vi "Send Message.vi"(4 "timeout in ms (100)":i32=100, 6 "Message ID":i32, 8 "error in (no error)":errorcluster, 9 "Data":variant, 10 "Command":string, 11 "RemoteControl.STM in":refnum<class "RemoteControl.STM.lvclass">) -> (0 "error out":errorcluster, 3 "RemoteControl.STM out":refnum<class "RemoteControl.STM.lvclass">)   [LabVIEW 2016, in "RemoteControl.STM.lvclass"]
uses:
  RemoteControl.STM.lvclass
  <vilib>/NI/STM/TCP/TCP Write Options.ctl
  RemoteControl/Typedefs/Variant with Message ID-cluster.ctl
  RemoteControl.STM.lvclass/RemoteControl.STM.ctl
  <vilib>/NI/STM/TCP/Write Message (TCP).vi
  <vilib>/NI/STM/NI STM.lvlib
  RemoteControl/RemoteControl.lvclass
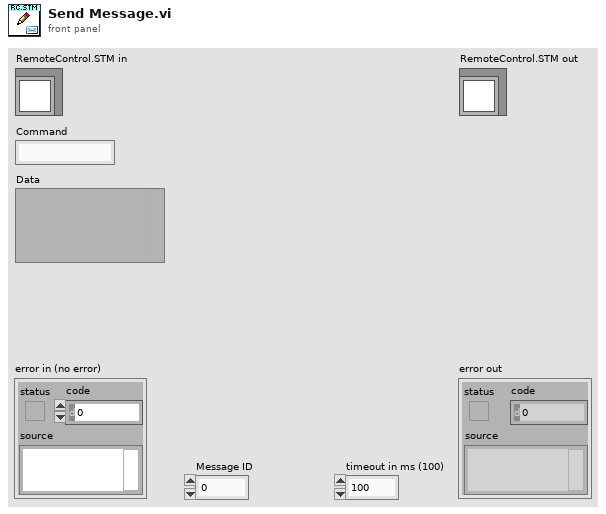
[diagram p1: front panel]
types:
  T1 = typedef "RemoteControl.lvclass/Variant with Message ID-cluster.ctl" = cluster{"Data":variant, "Message ID":i32}
  T2 = typedef "NI STM.lvlib/TCP Write Options.ctl" = cluster{"ignore timeout error":bool, "timeout ms (1000)":i32}
  T3 = typedef "NI STM.lvlib/TCP Connection Info.ctl" = cluster{"connection ID":refnum<k5>, "meta data":T4[]}
  T4 = typedef "NI STM.lvlib/MetaDataElement.ctl" = string
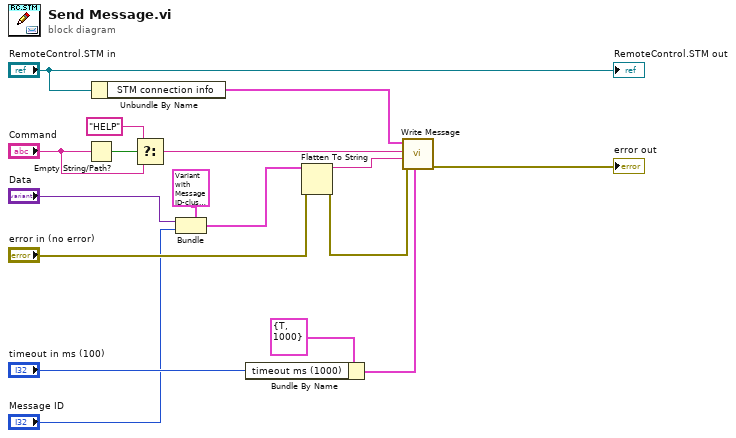
[diagram p0: block diagram]
diagram:
  n1 = Empty String/Path?(string/path="Command") -> (empty?=w8:bool)
  n2 = Unbundle By Name("RemoteControl.STM in") -> ("STM connection info"=w12:T3)
  n3 = Select(t="HELP", s=w8, f="Command") -> (s? t:f=w7:string)
  n4 = Bundle(cluster=T1 {"Data"=variant, "Message ID"=0} ("output cluster"), "Data"="Data", "Message ID"="Message ID") -> (w2:T1)
  n5 = Bundle By Name(cluster=T2 {"ignore timeout error"=TRUE, "timeout ms (1000)"=1000} ("options"), "timeout ms (1000)"="timeout in ms (100)") -> (w15:T2)
  n6 = Flatten To String(anything=w2, error in (no error)="error in (no error)") -> (data string=w17:string, error out=w9:errorcluster)  [unwired: 2 in, 1 out]
  n7 = call-poly <vilib>:"Write Message.vi"("options"=w15, "error in"=w9, "data"=w17, "name"=w7, "connection info in"=w12) -> ("error out"=→"error out":errorcluster)  [unwired: 5 in, 1 out]
  "RemoteControl.STM out" <- "RemoteControl.STM in"
